vi "change tag select name.vi"(8 "error in":errorcluster, 9 "new name":string, 10 "old name":string, 11 "tag select module configuration in":refnum<class "tag select module configuration.lvclass">) -> (0 "error out":errorcluster, 1 "changed channels":refnum<class "TBM channel.lvclass">[](array[class]), 3 "tag select module configuration out":refnum<class "tag select module configuration.lvclass">)   [LabVIEW 2013, in "tag select module configuration.lvclass"]
uses:
  tag select module configuration.lvclass
  <vilib>/NI/Tag Bus Module Framework/channel/TBM channel.lvclass
  tag select module configuration.lvclass/tag select module configuration.ctl
  <vilib>/NI/Tag Bus/tag/tag descriptor.lvclass/tag descriptor.ctl
  <vilib>/NI/Tag Bus/tag/tag descriptor.lvclass
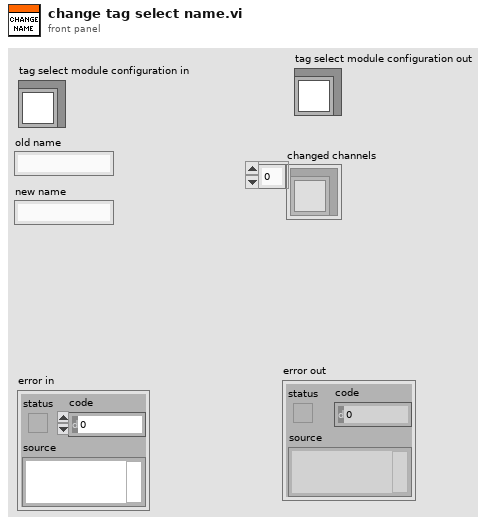
[diagram p1: front panel]
types:
  T1 = typedef "tag select module configuration.lvclass/tag select configuration.ctl" = cluster{"tag select name":string, "output":refnum<class "TBM channel.lvclass">, "select":refnum<class "TBM channel.lvclass">, "input channels":refnum<class "TBM channel.lvclass">[]}
  T2 = typedef "tag bus.lvlib/tag descriptor.lvclass/Data Type.ctl" = enum16{"Double", "Single", "I64", "I32", "I16", "I8", "U64", "U32", "U16", "U8", "Boolean", "String", "Array of Double", "Array of Single", "Array of I64", "Array of I32", "Array of I16", "Array of I8", "Array of U64", "Array of U32", "Array of U16", "Array of U8", "Array of Boolean", "Array of String"}
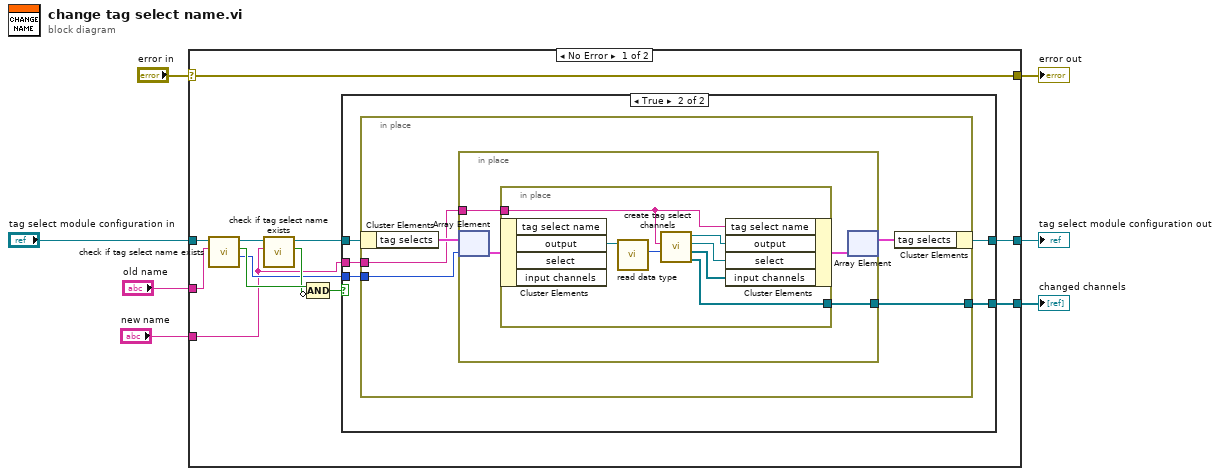
[diagram p0: block diagram]
diagram:
  n1 = case shown="No Error" "error in" {
    selector: "error in" -> [w19 w43]
    tunnel: [w19 w43] -> w6
    tunnel: [w16 w42] -> w4
    tunnel: "tag select module configuration in" -> [w18 w42]
    tunnel: "old name" -> [w17 _]
    tunnel: "new name" -> [w9 _]
    tunnel: [w8 _] -> w1
    frame No Error {
      n2 = call "check if tag select name exists.vi"("name to locate"=w17, "tag select module configuration in"=w18) -> ("index"=w10:i32, "found?"=w13:bool, "tag select module configuration out"=w15:refnum<class "tag select module configuration.lvclass">)  [unwired: 6 in, 1 out]
      n3 = call "check if tag select name exists.vi"("name to locate"=w9, "tag select module configuration in"=w15) -> ("found?"=w12:bool, "tag select module configuration out"=w14:refnum<class "tag select module configuration.lvclass">)  [unwired: 6 in, 2 out]
      n4 = Compound Arithmetic op=AND(w13, invert w12) -> (w11:bool)
      n5 = case shown="True" w11 {
        tunnel: w14 -> [w20 w25]
        tunnel: [w20 w24] -> w16
        tunnel: w10 -> [_ w23]
        tunnel: w9 -> [_ w22]
        tunnel: [_ w21] -> w8
        frame False {
        }
        frame True {
          n6 = in-place {
            in-place-border: w23 -> [w28]
            in-place-border: w22 -> [w27]
            in-place-border: [w26] -> w21
            n7 = in-place-cluster #1(w25) -> ("tag selects"=w30:T1[])
            n8 = in-place {
              in-place-border: w27 -> [w33]
              in-place-border: [w31] -> w26
              n9 = in-place-array #2(w30, w28) -> (w34:T1)
              n10 = in-place {
                in-place-border: w33 -> [w36]
                in-place-border: [w35] -> w31
                n11 = in-place-cluster #3(w34) -> ("output"=w41:refnum<class "TBM channel.lvclass">)  [unwired: 3 out]
                n12 = call <vilib>:"read data type.vi"("system tag in"=w41) -> ("data type"=w40:T2)  [unwired: 8 in, 2 out]
                n13 = call "create tag select channels.vi"("data type"=w40, "tag select name"=w36) -> ("created channels"=w35:refnum<class "TBM channel.lvclass">[], "inputs"=w37:refnum<class "TBM channel.lvclass">[], "select"=w38:refnum<class "TBM channel.lvclass">, "output"=w39:refnum<class "TBM channel.lvclass">)  [unwired: 6 in]
                n14 = in-place-cluster #3("tag select name"=w36, "output"=w39, "select"=w38, "input channels"=w37) -> (w32:T1)
              }
              n15 = in-place-array #2(w32) -> (w29:T1[])  [unwired: 1 out]
            }
            n16 = in-place-cluster #1("tag selects"=w29) -> (w24:refnum<class "tag select module configuration.lvclass">)
          }
        }
      }
    }
    frame Error {
    }
  }
  "error out" <- w6
  "tag select module configuration out" <- w4
  "changed channels" <- w1
